vi "Escape Regexp String.vi"(11 "Input":string) -> (3 "Escaped Regexp String":string)   [LabVIEW 2020, in "Stream.lvlib" / "URLPattern.lvclass"]
uses:
  URLPattern.lvclass
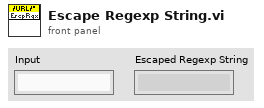
[diagram p1: front panel]
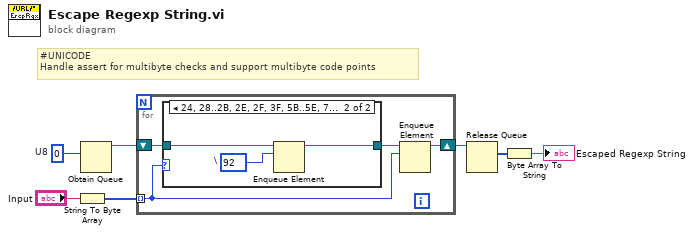
[diagram p0: block diagram]
diagram:
  w6 = u8 0  # U8
  # "#UNICODE\nHandle assert for multibyte checks and support multibyte code points"
  n1 = String To Byte Array(string="Input") -> (unsigned byte array=w5:u8[])
  n2 = Obtain Queue(element data type=w6) -> (queue out=w4:refnum<queue>)  [unwired: 4 in, 2 out]
  n3 = for {
    tunnel: w5 -> [w9] mode=indexing
    shift-right: [w8] -> w3
    shift-left: w4 -> [w11]
    n4 = case shown="24, 28..2B, 2E, 2F, 3F, 5B..5E, 7B..7D" w9 {
      tunnel: w11 -> [w12 w15]
      tunnel: [w12 w13] -> w10
      frame Default {
      }
      frame 36, 40..43, 46, 47, 63, 91..94, 123..125 {
        w14 = u8 92  # \
        n5 = Enqueue Element(queue=w15, element=w14) -> (queue out=w13:refnum<queue>)  [unwired: 2 in, 2 out]
      }
    }
    n6 = Enqueue Element(queue=w10, element=w9) -> (queue out=w8:refnum<queue>)  [unwired: 2 in, 2 out]
  }
  n7 = Release Queue(queue=w3) -> (remaining elements=w2:u8[])  [unwired: 2 in, 2 out]
  n8 = Byte Array To String(unsigned byte array=w2) -> (string=→"Escaped Regexp String":string)
